vi "Emballage_BDD_enregistrement_SQL.vi"(5 "SN_PRODUIT":string, 6 "NO_DU_CARTON":i32, 7 "NO_RETOUR_CLIENT":string, 8 "entrée d'erreur":errorcluster, 9 "NO_CDEVAL":string, 10 "ID_ARTICLE_GPAO":string, 11 "ID_UTILISATEUR_GPAO":string) -> (0 "sortie d'erreur":errorcluster)   [LabVIEW 2020]
uses:
  Modules/FS/60_FS_Controles/60_FS_SetGet.ctl
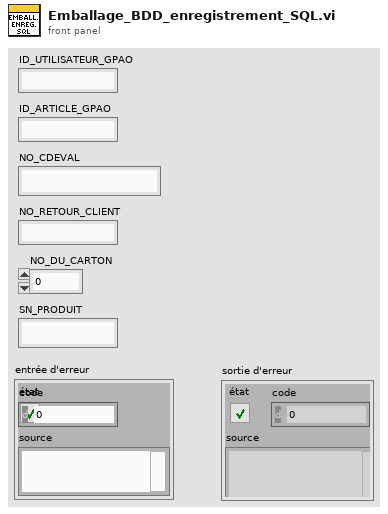
[diagram p1: front panel]
types:
  T1 = typedef "60_FS_SetGet.ctl" = enum16{"set", "get"}
  T2 = typedef "60_FS_CLT_Chemins.ctl" = cluster{"Racine_local":path, "Racine_reseau":path, "Racine_Support_Application":path, "Fichier_Journalisation":path, "Connexion_BDD_VSX":path, "Connexion_BDD_PLZ":path}
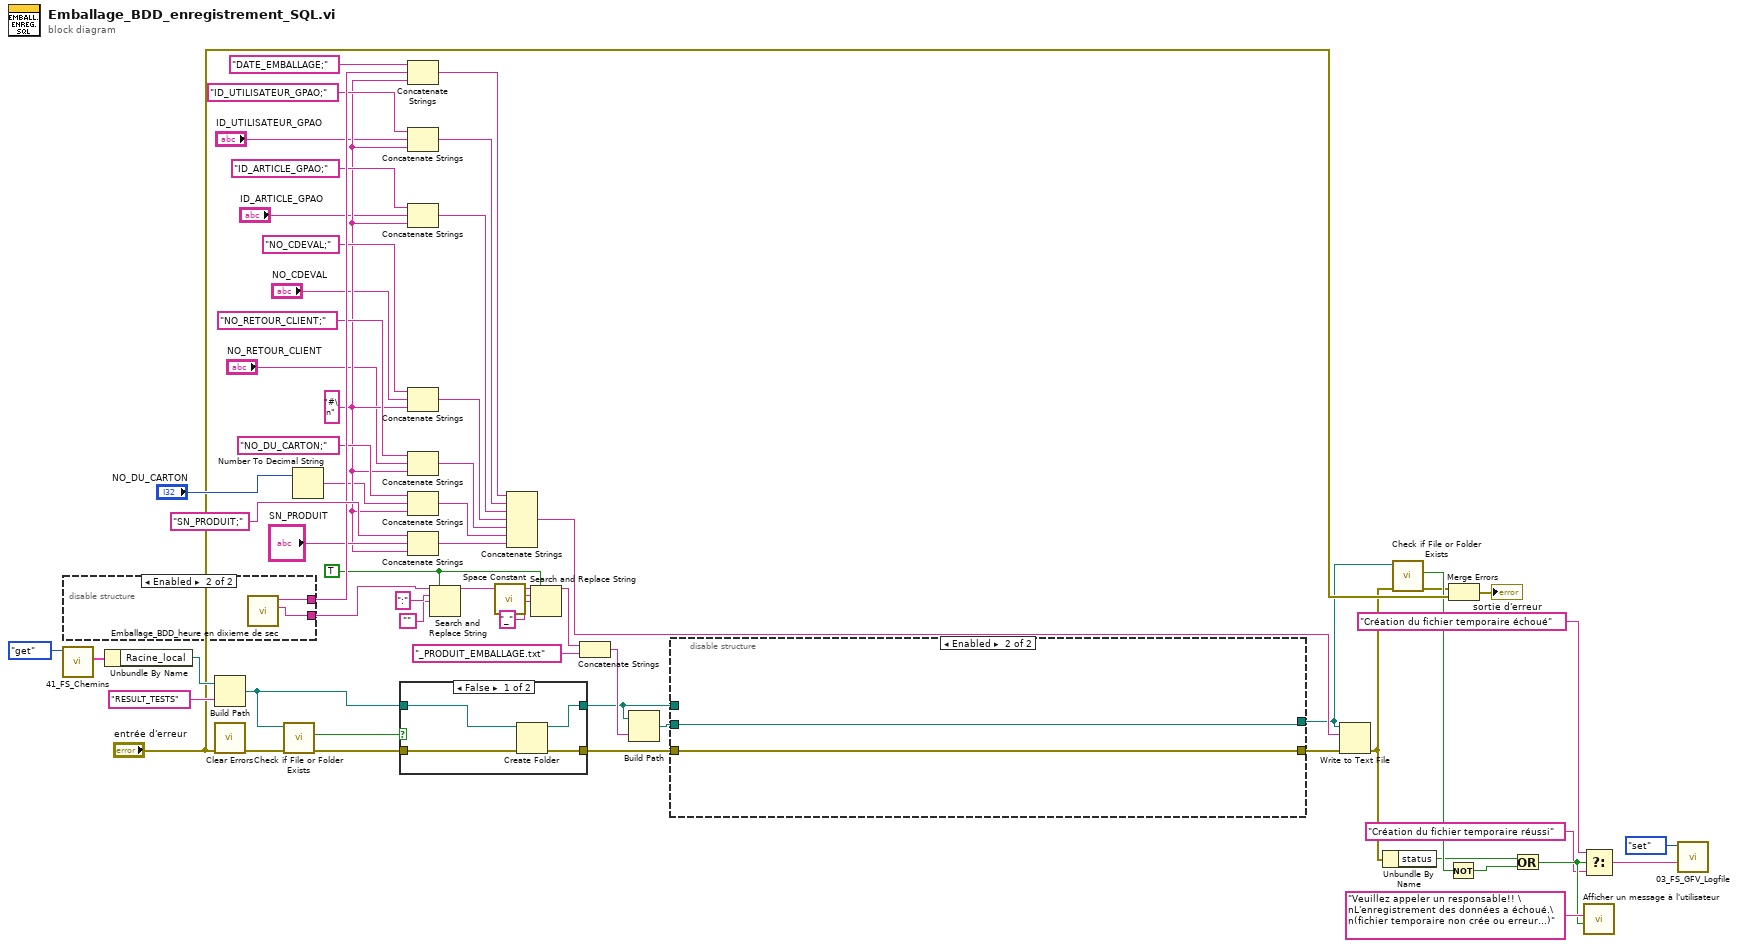
[diagram p0: block diagram]
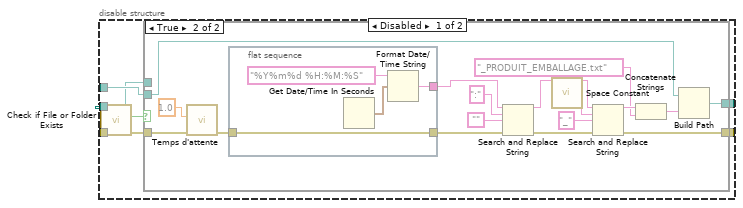
[diagram p2: hidden frame]
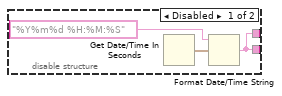
[diagram p4: hidden frame]
diagram:
  w47 = TRUE ("tout remplacer ? (F)")
  w33 = "#\n"
  n1 = call "41_FS_Chemins.vi"("SetGet"=60_FS_SetGet."get") -> ("CLT_Chemins_out"=w27:T2)  [unwired: 9 in, 1 out]
  n2 = disable-structure shown="Enabled" {
    disable-tunnel: [w61 w64] -> w48
    disable-tunnel: [w61 w65] -> w1
    frame Disabled {
      n3 = Get Date/Time In Seconds() -> (seconds since 1Jan1904=w62:timestamp)
      n4 = Format Date/Time String(time format string (%c)="%Y%m%d %H:%M:%S" ("chaîne de format de l'heure (%c)"), seconds (now)=w62) -> (date/time string=w61:string)  [unwired: 1 in]
    }
    frame Enabled {
      n5 = call "Emballage_BDD_heure en dixieme de sec.vi"() -> ("chaîne de date/heure avec dixieme de sec"=w65:string, "chaîne de date/heure"=w64:string)  [unwired: 10 in]
    }
  }
  n6 = Unbundle By Name(w27) -> ("Racine_local"=w26:path)
  n7 = Build Path(base path=w26, name or relative path="RESULT_TESTS" ("chemin de base")) -> (appended path=w20:path)
  n8 = call <vilib>:"Clear Errors.vi"("error in (no error)"="entrée d'erreur") -> ("error out"=w17:errorcluster)  [unwired: 5 in, 1 out]
  n9 = call <vilib>:"Check if File or Folder Exists.vi"("error in (no error)"=w17, "path"=w20) -> ("error out"=w21:errorcluster, "file or folder exists?"=w22:bool)  [unwired: 7 in, 1 out]
  n10 = Number To Decimal String(number="NO_DU_CARTON") -> (decimal integer string=w28:string)  [unwired: 1 in]
  n11 = case shown="False" w22 {
    tunnel: w20 -> [w69 w71]
    tunnel: [w68 w71] -> w5
    tunnel: w21 -> [w67 w70]
    tunnel: [w66 w70] -> w6
    frame False {
      n12 = Create Folder(path (use dialog)=w69, error in=w67) -> (created path=w68:path, error out=w66:errorcluster)  [unwired: 1 in, 1 out]
    }
    frame True {
    }
  }
  n13 = Concatenate Strings("DATE_EMBALLAGE;" ("chaîne"), w48, w33) -> (w41:string)
  n14 = Concatenate Strings("ID_UTILISATEUR_GPAO;" ("chaîne"), "ID_UTILISATEUR_GPAO", w33) -> (w39:string)
  n15 = Concatenate Strings("ID_ARTICLE_GPAO;" ("chaîne"), "ID_ARTICLE_GPAO", w33) -> (w37:string)
  n16 = Concatenate Strings("NO_CDEVAL;" ("chaîne"), "NO_CDEVAL", w33) -> (w34:string)
  n17 = Concatenate Strings("NO_RETOUR_CLIENT;" ("chaîne"), "NO_RETOUR_CLIENT", w33) -> (w40:string)
  n18 = Concatenate Strings("NO_DU_CARTON;" ("chaîne"), w28, w33) -> (w38:string)
  n19 = Concatenate Strings("SN_PRODUIT;" ("chaîne"), "SN_PRODUIT", w33) -> (w57:string)
  n20 = Search and Replace String(replace all?=w47, input string=w1, search string=":" ("chaîne recherchée"), replace string="") -> (result string=w52:string)  [unwired: 4 in, 3 out]
  n21 = call <vilib>:"Space Constant.vi"() -> ("String"=w51:string)
  n22 = Concatenate Strings(w41, w39, w37, w34, w40, w38, w57) -> (w46:string)
  n23 = Search and Replace String(replace all?=w47, input string=w52, search string=w51, replace string="_" ("chaîne de remplacement (\"\")")) -> (result string=w49:string)  [unwired: 4 in, 3 out]
  n24 = Concatenate Strings(w49, "_PRODUIT_EMBALLAGE.txt" ("chaîne")) -> (w56:string)
  n25 = Build Path(base path=w5, name or relative path=w56) -> (appended path=w3:path)
  n26 = disable-structure shown="Enabled" {
    disable-tunnel: w6 -> [w78 w103]
    disable-tunnel: w5 -> [w76 _]
    disable-tunnel: [w75 w102] -> w4
    disable-tunnel: w3 -> [w74 w102]
    disable-tunnel: [w72 w103] -> w2
    frame Disabled {
      n27 = call <vilib>:"Check if File or Folder Exists.vi"("error in (no error)"=w78, "path"=w74) -> ("error out"=w73:errorcluster, "file or folder exists?"=w77:bool)  [unwired: 7 in, 1 out]
      n28 = case shown="True" w77 {
        tunnel: w76 -> [_ w88]
        tunnel: [w80 w87] -> w75
        tunnel: w74 -> [w80 _]
        tunnel: w73 -> [w79 w86]
        tunnel: [w79 w82] -> w72
        frame False {
        }
        frame True {
          n29 = call "Temps d'attente"("error in (no error)"=w86, "Delay Time (s)"=1.0) -> ("error out"=w84:errorcluster)  [unwired: 9 in]
          n30 = flat-sequence {
            tunnel: [w99] -> w89
            tunnel: [w98] -> w85
            tunnel: w84 -> [w98]
            frame #0 {
              n31 = Get Date/Time In Seconds() -> (seconds since 1Jan1904=w101:timestamp)
              n32 = Format Date/Time String(time format string (%c)="%Y%m%d %H:%M:%S" ("chaîne de format de l'heure (%c)"), seconds (now)=w101) -> (date/time string=w99:string)  [unwired: 1 in]
            }
          }
          n33 = Search and Replace String(input string=w89, search string=":" ("chaîne recherchée"), replace string="", error in=w85) -> (result string=w94:string, error out=w83:errorcluster)  [unwired: 4 in, 2 out]
          n34 = call <vilib>:"Space Constant.vi"() -> ("String"=w95:string)
          n35 = Search and Replace String(input string=w94, search string=w95, replace string="_" ("chaîne de remplacement (\"\")"), error in=w83) -> (result string=w97:string, error out=w82:errorcluster)  [unwired: 4 in, 2 out]
          n36 = Concatenate Strings(w97, "_PRODUIT_EMBALLAGE.txt" ("chaîne")) -> (w90:string)
          n37 = Build Path(base path=w88, name or relative path=w90) -> (appended path=w87:path)
        }
      }
    }
    frame Enabled {
    }
  }
  n38 = Write to Text File(file (use dialog)=w4, text=w46, error in=w2) -> (error out=w12:errorcluster)  [unwired: 1 in, 2 out]
  n39 = Unbundle By Name(w12) -> ("status"=w13:bool)
  n40 = call <vilib>:"Check if File or Folder Exists.vi"("error in (no error)"=w12, "path"=w4) -> ("error out"=w14:errorcluster, "file or folder exists?"=w16:bool)  [unwired: 7 in, 1 out]
  n41 = Not(x=w16) -> (.not. x?=w15:bool)
  n42 = Merge Errors(w14, "entrée d'erreur") -> (→"sortie d'erreur":errorcluster)
  n43 = Or(x=w13, y=w15) -> (x .or. y?=w9:bool)
  n44 = Select(t="Création du fichier temporaire échoué", s=w9, f="Création du fichier temporaire réussi") -> (s? t:f=w10:string)
  n45 = call "Afficher un message à l'utilisateur"("Enable"=w9, "Message"="Veuillez appeler un responsable!! \nL'enregistrement des données a échoué.\n(fichier temporaire non crée ou erreur...)") -> ()  [unwired: 8 in, 2 out]
  n46 = call "03_FS_GFV_Logfile.vi"("Chaîne"=w10, "States"=60_FS_SetGet."set") -> ()  [unwired: 8 in, 2 out]
